vi "TestJComplete.vi"() -> ()   [LabVIEW 2009]
panel:
  in  "file path (use dialog)":path
  in  "FPGA IP Address":string
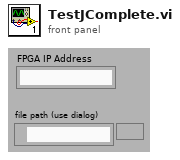
[diagram p1: front panel]
types:
  T1 = enum16{"open", "replace", "create", "open or create", "replace or create", "replace or create with confirmation"}
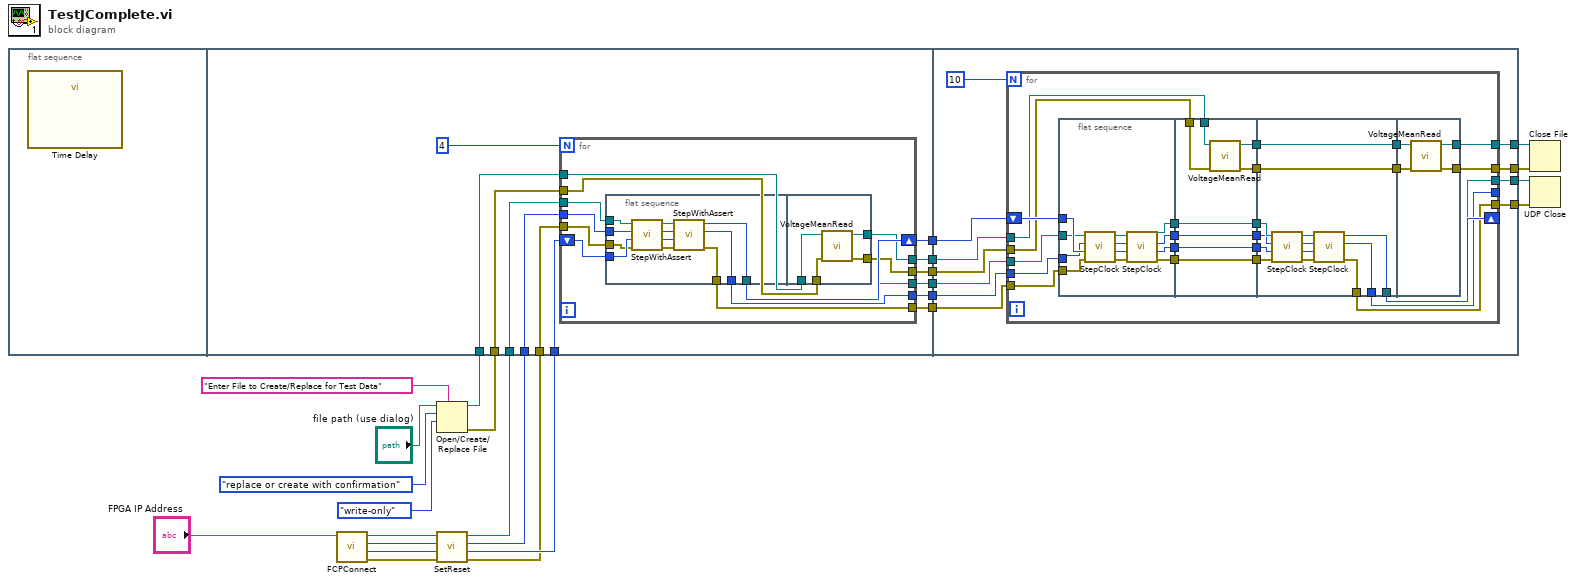
[diagram p0: block diagram]
diagram:
  n1 = flat-sequence {
    tunnel: w7 -> [w32]
    tunnel: w8 -> [w33]
    tunnel: w9 -> [w34]
    tunnel: w10 -> [w35]
    tunnel: w11 -> [w36]
    tunnel: w12 -> [w37]
    tunnel: [w31] -> w6
    tunnel: [w30] -> w5
    tunnel: [w29] -> w4
    tunnel: [w28] -> w3
    tunnel: [w27] -> w2
    tunnel: [w26] -> w1
    tunnel: [w76] -> w20
    tunnel: [w75] -> w19
    tunnel: [w74] -> w14
    tunnel: [w73] -> w13
    tunnel: w6 -> [w72]
    tunnel: w5 -> [w71]
    tunnel: w4 -> [w70]
    tunnel: w3 -> [w69]
    tunnel: w2 -> [w68]
    tunnel: w1 -> [w67]
    frame #0 {
      n2 = call "Time Delay"() -> ()  [unwired: 11 in, 1 out]
    }
    frame #1 {
      n3 = for {
        N: 4 -> [_]
        tunnel: w37 -> [w50]
        tunnel: w36 -> [w49]
        shift-right: [w46] -> w28
        shift-left: w35 -> [w48]
        tunnel: w34 -> [w47]
        tunnel: w33 -> [w45]
        tunnel: w32 -> [w44]
        tunnel: [w43] -> w31
        tunnel: [w42] -> w30
        tunnel: [w41] -> w29
        tunnel: [w40] -> w27
        tunnel: [w39] -> w26
        n4 = flat-sequence {
          tunnel: w50 -> [w62]
          tunnel: w49 -> [w61]
          tunnel: w48 -> [w60]
          tunnel: w47 -> [w59]
          tunnel: [w54] -> w46
          tunnel: [w53] -> w43
          tunnel: [w52] -> w42
          tunnel: [w51] -> w41
          tunnel: w45 -> [w66]
          tunnel: w44 -> [w65]
          tunnel: [w64] -> w40
          tunnel: [w63] -> w39
          frame #0 {
            n5 = call "StepWithAssert.vi"("error in (no error)"=w59, "SequenceNumber"=w60, "address"=w61, "connection ID"=w62) -> ("error out"=w55:errorcluster, "SequenceNumber out"=w56:i32, "address out"=w57:u32, "connection ID out"=w58:refnum<k16>)  [unwired: 4 in]
            n6 = call "StepWithAssert.vi"("error in (no error)"=w55, "SequenceNumber"=w56, "address"=w57, "connection ID"=w58) -> ("error out"=w51:errorcluster, "SequenceNumber out"=w54:i32, "address out"=w52:u32, "connection ID out"=w53:refnum<k16>)  [unwired: 4 in]
          }
          frame #1 {
            n7 = call "VoltageMeanRead.vi"("error in"=w65, "refnum"=w66) -> ("error out"=w63:errorcluster, "refnum out"=w64:refnum<file>)  [unwired: 8 in]
          }
        }
      }
    }
    frame #2 {
      n8 = for {
        N: 10 -> [_]
        tunnel: [w88] -> w76
        tunnel: [w87] -> w75
        shift-right: [w89] -> _
        shift-left: w69 -> [w101]
        tunnel: [w79] -> w74
        tunnel: [w78] -> w73
        tunnel: w72 -> [w100]
        tunnel: w71 -> [w99]
        tunnel: w70 -> [w98]
        tunnel: [w86] -> _
        tunnel: w68 -> [w85]
        tunnel: w67 -> [w84]
        n9 = flat-sequence {
          tunnel: w101 -> [w113]
          tunnel: w100 -> [w112]
          tunnel: w99 -> [w111]
          tunnel: w98 -> [w110]
          tunnel: [w105] -> w96
          tunnel: [w104] -> w94
          tunnel: [w103] -> w92
          tunnel: [w102] -> w90
          tunnel: [w121] -> w97
          tunnel: w96 -> [w121]
          tunnel: [w120] -> w95
          tunnel: w94 -> [w120]
          tunnel: [w119] -> w93
          tunnel: w92 -> [w119]
          tunnel: [w118] -> w91
          tunnel: w90 -> [w118]
          tunnel: w85 -> [w117]
          tunnel: w84 -> [w116]
          tunnel: [w115] -> w82
          tunnel: [w114] -> w80
          tunnel: w97 -> [w135]
          tunnel: w95 -> [w134]
          tunnel: w93 -> [w133]
          tunnel: w91 -> [w132]
          tunnel: [w127] -> w89
          tunnel: [w126] -> w88
          tunnel: [w125] -> w87
          tunnel: [w124] -> w86
          tunnel: [w123] -> w83
          tunnel: w82 -> [w123]
          tunnel: [w122] -> w81
          tunnel: w80 -> [w122]
          tunnel: w83 -> [w139]
          tunnel: w81 -> [w138]
          tunnel: [w137] -> w79
          tunnel: [w136] -> w78
          frame #0 {
            n10 = call "StepClock.vi"("error in (no error)"=w110, "SequenceNumber"=w113, "address"=w111, "connection ID"=w112) -> ("error out"=w106:errorcluster, "SequenceNumber out"=w107:i32, "address out"=w108:u32, "connection ID out"=w109:refnum<k16>)  [unwired: 4 in]
            n11 = call "StepClock.vi"("error in (no error)"=w106, "SequenceNumber"=w107, "address"=w108, "connection ID"=w109) -> ("error out"=w102:errorcluster, "SequenceNumber out"=w103:i32, "address out"=w104:u32, "connection ID out"=w105:refnum<k16>)  [unwired: 4 in]
          }
          frame #1 {
            n12 = call "VoltageMeanRead.vi"("error in"=w116, "refnum"=w117) -> ("error out"=w114:errorcluster, "refnum out"=w115:refnum<file>)  [unwired: 8 in]
          }
          frame #2 {
            n13 = call "StepClock.vi"("error in (no error)"=w132, "SequenceNumber"=w133, "address"=w134, "connection ID"=w135) -> ("error out"=w128:errorcluster, "SequenceNumber out"=w129:i32, "address out"=w130:u32, "connection ID out"=w131:refnum<k16>)  [unwired: 4 in]
            n14 = call "StepClock.vi"("error in (no error)"=w128, "SequenceNumber"=w129, "address"=w130, "connection ID"=w131) -> ("error out"=w125:errorcluster, "SequenceNumber out"=w127:i32, "address out"=w124:u32, "connection ID out"=w126:refnum<k16>)  [unwired: 4 in]
          }
          frame #3 {
            n15 = call "VoltageMeanRead.vi"("error in"=w138, "refnum"=w139) -> ("error out"=w136:errorcluster, "refnum out"=w137:refnum<file>)  [unwired: 8 in]
          }
        }
      }
    }
  }
  n16 = call "FCPConnect.vi"("FPGA IP Address"="FPGA IP Address") -> ("error out"=w23:errorcluster, "Sequence Number"=w21:i32, "FPGA IP Address Out"=w22:u32, "connection ID out"=w24:refnum<k16>)  [unwired: 7 in]
  n17 = Open/Create/Replace File(file path (use dialog)="file path (use dialog)", prompt="Enter File to Create/Replace for Test Data", operation (0:open)=T1."replace or create with confirmation", access (0:read/write)=enum16{"read/write", "read-only", "write-only"}."write-only") -> (refnum out=w8:refnum<file>, error out=w7:errorcluster)  [unwired: 2 in, 1 out]
  n18 = call "SetReset.vi"("error in (no error)"=w23, "SequenceNumber"=w21, "address"=w22, "connection ID"=w24) -> ("error out"=w9:errorcluster, "SequenceNumber out"=w10:i32, "Address out"=w11:u32, "connection ID out"=w12:refnum<k16>)  [unwired: 4 in]
  n19 = Close File(refnum=w14, error in=w13) -> ()  [unwired: 2 out]
  n20 = UDP Close(connection ID=w20, 8:w19) -> ()  [unwired: 2 out]
